vi "Skew_Image5.vi"(4 "[IN] Skewed Image":T1, 5 "[IN] Share Angle":u16 max=89 step=1, 6 "[IN] Calculation mode":enum16{"Single core", "2x cores", "4x cores"}(ring), 7 "error IN":errorcluster, 8 "[IN] Y = Array rows":i32, 9 "[IN] X = Array cols":i32, 10 "[IN] Source Image U16":u16[][](array[numeric])) -> (0 "error OUT":errorcluster, 3 "[OUT] Skewed Image":T1)   [LabVIEW 2020]
uses:
  <vilib>/vision/Image Controls.llb/IMAQ Image.ctl
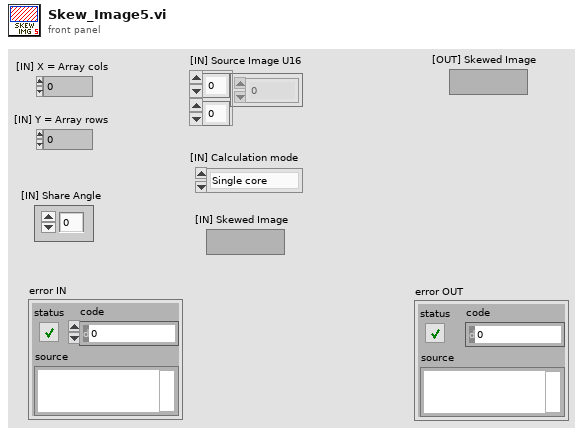
[diagram p1: front panel]
types:
  T1 = typedef "IMAQ Image.ctl" = refnum<image>
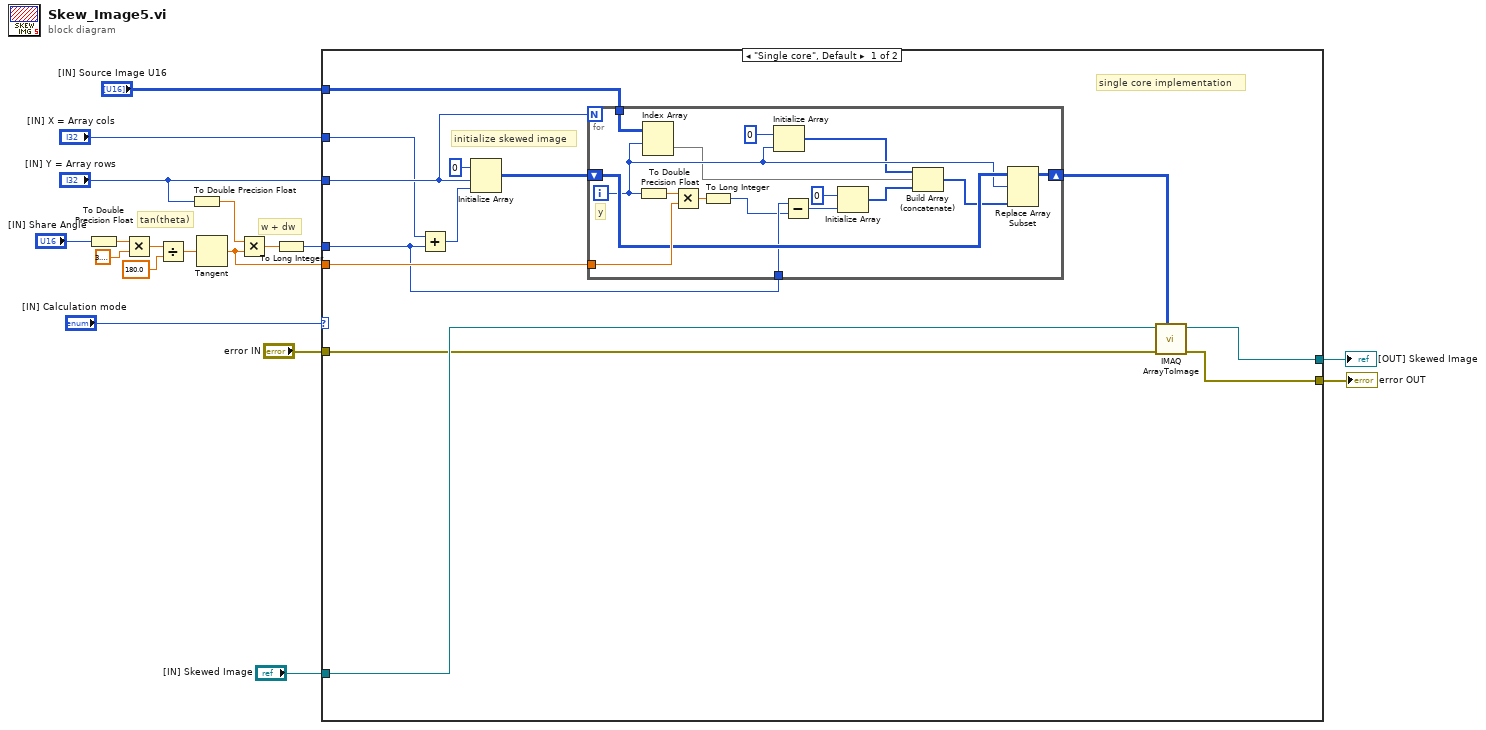
[diagram p0: block diagram]
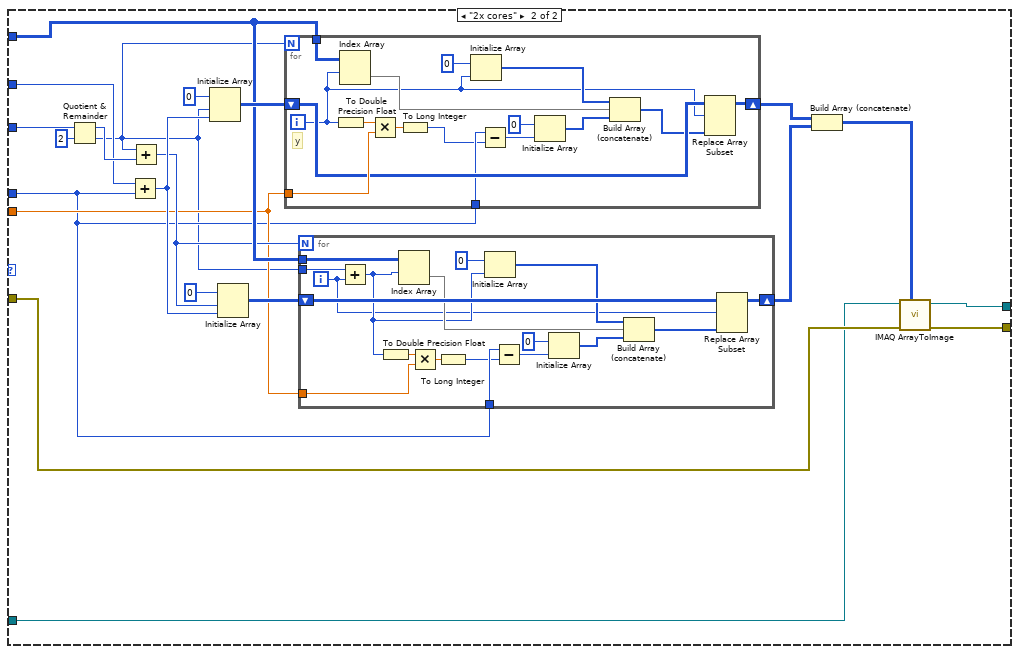
[diagram p2: hidden frame]
diagram:
  # "w + dw"
  # "tan(theta)"
  n1 = To Double Precision Float(number="[IN] Share Angle") -> (double precision float=w18:dbl)
  n2 = Multiply(x=w18, y=3.141592653589793) -> (x*y=w17:dbl)
  n3 = Divide(x=w17, y=180.0) -> (x/y=w15:dbl)
  n4 = To Double Precision Float(number="[IN] Y = Array rows") -> (double precision float=w9:dbl)
  n5 = Tangent(1:w15) -> (0:w13:dbl)
  n6 = Multiply(x=w9, y=w13) -> (x*y=w12:dbl)
  n7 = To Long Integer(number=w12) -> (32bit integer=w14:i32)
  n8 = case shown="\"Single core\", Default" "[IN] Calculation mode" {
    tunnel: w14 -> [w19 w56]
    tunnel: w13 -> [w27 w57]
    tunnel: "[IN] Source Image U16" -> [w24 w59]
    tunnel: "[IN] X = Array cols" -> [w25 w63]
    tunnel: "[IN] Y = Array rows" -> [w26 w62]
    tunnel: "error IN" -> [w20 w52]
    tunnel: [w22 w51] -> w4
    tunnel: [w21 w50] -> w3
    tunnel: "[IN] Skewed Image" -> [w31 w49]
    frame "Single core", Default {
      # "single core implementation"
      # "initialize skewed image"
      n9 = Add(x=w25, y=w19) -> (x+y=w29:i32)
      n10 = Initialize Array(u16 0, w26, w29) -> (w28:u16[][])
      n11 = for {
        N: w26 -> [_]
        shift-right: [w42] -> w23
        shift-left: w28 -> [w43]
        tunnel: w24 -> [w47]
        tunnel: w27 -> [w45]
        tunnel: w19 -> [w39]
        i -> [w40]
        # "y"
        n12 = To Double Precision Float(number=w40) -> (double precision float=w46:dbl)
        n13 = Index Array(array=w47, index (row)=w40) -> (element=w34:u16[])  [unwired: 1 in]
        n14 = Multiply(x=w46, y=w45) -> (x*y=w44:dbl)
        n15 = To Long Integer(number=w44) -> (32bit integer=w38:i32)
        n16 = Initialize Array(u16 0, w40) -> (w35:u16[])
        n17 = Subtract(x=w39, y=w38) -> (x-y=w36:i32)
        n18 = Initialize Array(u16 0, w36) -> (w33:u16[])
        n19 = Build Array (concatenate)(w35, w34, w33) -> (w32:u16[])
        n20 = Replace Array Subset(array=w43, new element=w32, index (row)=w40) -> (w42:u16[][])  [unwired: 1 in]
      }
      n21 = call "IMAQ ArrayToImage"("Image Pixels (U16)"=w23, "error in (no error)"=w20, "Image"=w31) -> ("error out"=w22:errorcluster, "Image Out"=w21:T1)  [unwired: 7 in]
    }
    frame "2x cores" {
      n22 = Quotient & Remainder(x=w62, y=2) -> (x-y*floor(x/y)=w66:i32, floor(x/y)=w48:i32)
      n23 = Add(x=w63, y=w56) -> (x+y=w64:i32)
      n24 = Add(x=w48, y=w66) -> (x+y=w58:i32)
      n25 = Initialize Array(u16 0, w48, w64) -> (w61:u16[][])
      n26 = Initialize Array(u16 0, w58, w64) -> (w60:u16[][])
      n27 = for {
        N: w48 -> [_]
        shift-right: [w97] -> w55
        shift-left: w61 -> [w98]
        tunnel: w59 -> [w102]
        tunnel: w57 -> [w100]
        tunnel: w56 -> [w95]
        i -> [w87]
        # "y"
        n28 = To Double Precision Float(number=w87) -> (double precision float=w101:dbl)
        n29 = Index Array(array=w102, index (row)=w87) -> (element=w90:u16[])  [unwired: 1 in]
        n30 = Multiply(x=w101, y=w100) -> (x*y=w99:dbl)
        n31 = To Long Integer(number=w99) -> (32bit integer=w94:i32)
        n32 = Initialize Array(u16 0, w87) -> (w91:u16[])
        n33 = Subtract(x=w95, y=w94) -> (x-y=w92:i32)
        n34 = Initialize Array(u16 0, w92) -> (w89:u16[])
        n35 = Build Array (concatenate)(w91, w90, w89) -> (w88:u16[])
        n36 = Replace Array Subset(array=w98, new element=w88, index (row)=w87) -> (w97:u16[][])  [unwired: 1 in]
      }
      n37 = for {
        N: w58 -> [_]
        shift-right: [w81] -> w54
        shift-left: w60 -> [w82]
        tunnel: w59 -> [w86]
        tunnel: w57 -> [w84]
        tunnel: w56 -> [w79]
        tunnel: w48 -> [w71]
        i -> [w69]
        n38 = Add(x=w71, y=w69) -> (x+y=w70:i32)
        n39 = To Double Precision Float(number=w70) -> (double precision float=w85:dbl)
        n40 = Index Array(array=w86, index (row)=w70) -> (element=w74:u16[])  [unwired: 1 in]
        n41 = Multiply(x=w85, y=w84) -> (x*y=w83:dbl)
        n42 = To Long Integer(number=w83) -> (32bit integer=w78:i32)
        n43 = Initialize Array(u16 0, w70) -> (w75:u16[])
        n44 = Subtract(x=w79, y=w78) -> (x-y=w76:i32)
        n45 = Initialize Array(u16 0, w76) -> (w73:u16[])
        n46 = Build Array (concatenate)(w75, w74, w73) -> (w72:u16[])
        n47 = Replace Array Subset(array=w82, new element=w72, index (row)=w69) -> (w81:u16[][])  [unwired: 1 in]
      }
      n48 = Build Array (concatenate)(w55, w54) -> (w53:u16[][])
      n49 = call "IMAQ ArrayToImage"("Image Pixels (U16)"=w53, "error in (no error)"=w52, "Image"=w49) -> ("error out"=w51:errorcluster, "Image Out"=w50:T1)  [unwired: 7 in]
    }
  }
  "error OUT" <- w4
  "[OUT] Skewed Image" <- w3
